vi "MEASURE_hysteresis - test.vi"() -> ()   [LabVIEW 2020]
uses:
  <vilib>/Utility/file.llb/Write To Spreadsheet File (DBL).vi
  <instrlib>/Keithley 24XX/Keithley 24XX.lvlib
panel:
  in  "Parameter":u16(ring)=1 items=["X", "Y", "R", "Theta", "Xh1", "Yh1", "Rh1", "Theta h1", "Xh2", "Yh2", "Rh2", "Theta h2", "Noise", "A1", "A2", "A3", "A4", "Frequency"]
  in  "harmonic 1":u8
  in  "Manual Phase":dbl=0.05
  in  "Sine Output Amplitude (1 V) 2":dbl=0.05
  in  "Input Connection (0: Single-Ended)":u16(ring) items=["Single-Ended Voltage", "Differential Voltage", "1 MOhm Current Gain", "100 MOhm Current Gain"]
  in  "frequency":dbl=50.0 format="%#_13g"
  out "loop run":i32
  in  "loop #":i32
  in  "Save data or not":bool=TRUE
  in  "path (folder + filename)":string="D:\\Kedar\\MoS2\\jw7_DJ_bulk_111213\\VvsHtr\\VvsHtr_300K"
  in  "Clear Plot":bool
  out "XY Graph":cluster{dbl[], dbl[]}(graph)
  out "LOCKIN Measurement":dbl
  out "gate voltage":dbl format="%#_13g"
  out "gate leaking":string="defbuffer1"
  in  "GATE STEP(mv)":i32
  in  "GATE Low Value (default 0)":dbl=1.0
  in  "GATE High Value":dbl=1.0
  in  "Function (0: Volts) 2":u16(ring) items=["Volts", "Current", "Resistance"]
  in  "Source Compaliance":dbl=1e-06
  in  "V address":refnum<visa-resource-name>="GPIB0::24::INSTR"
  in  "SD stabilization(S) 2":dbl format="%#_13g"
  in  "GATE / SD stablization 3":dbl format="%#_13g"
  in  "LOCKIN address":refnum<visa-resource-name>="GPIB0::24::INSTR"
  # "Lock-in"
  # "Gate Setting"
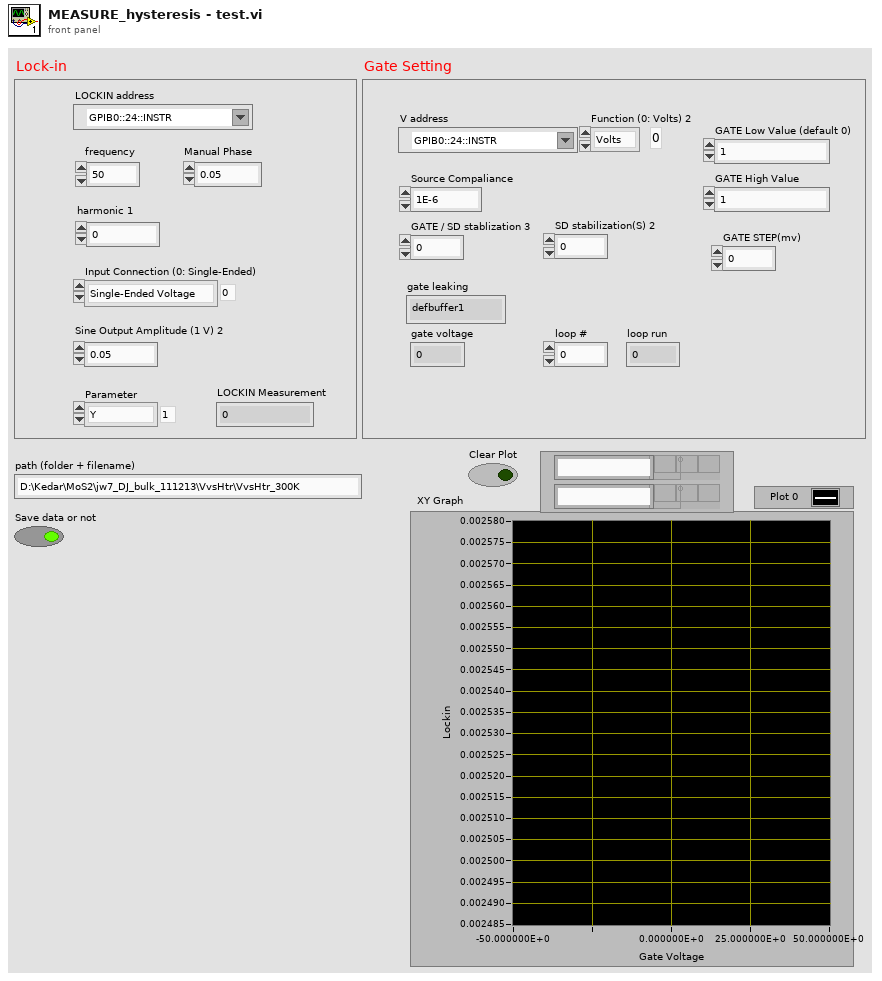
[diagram p1: front panel]
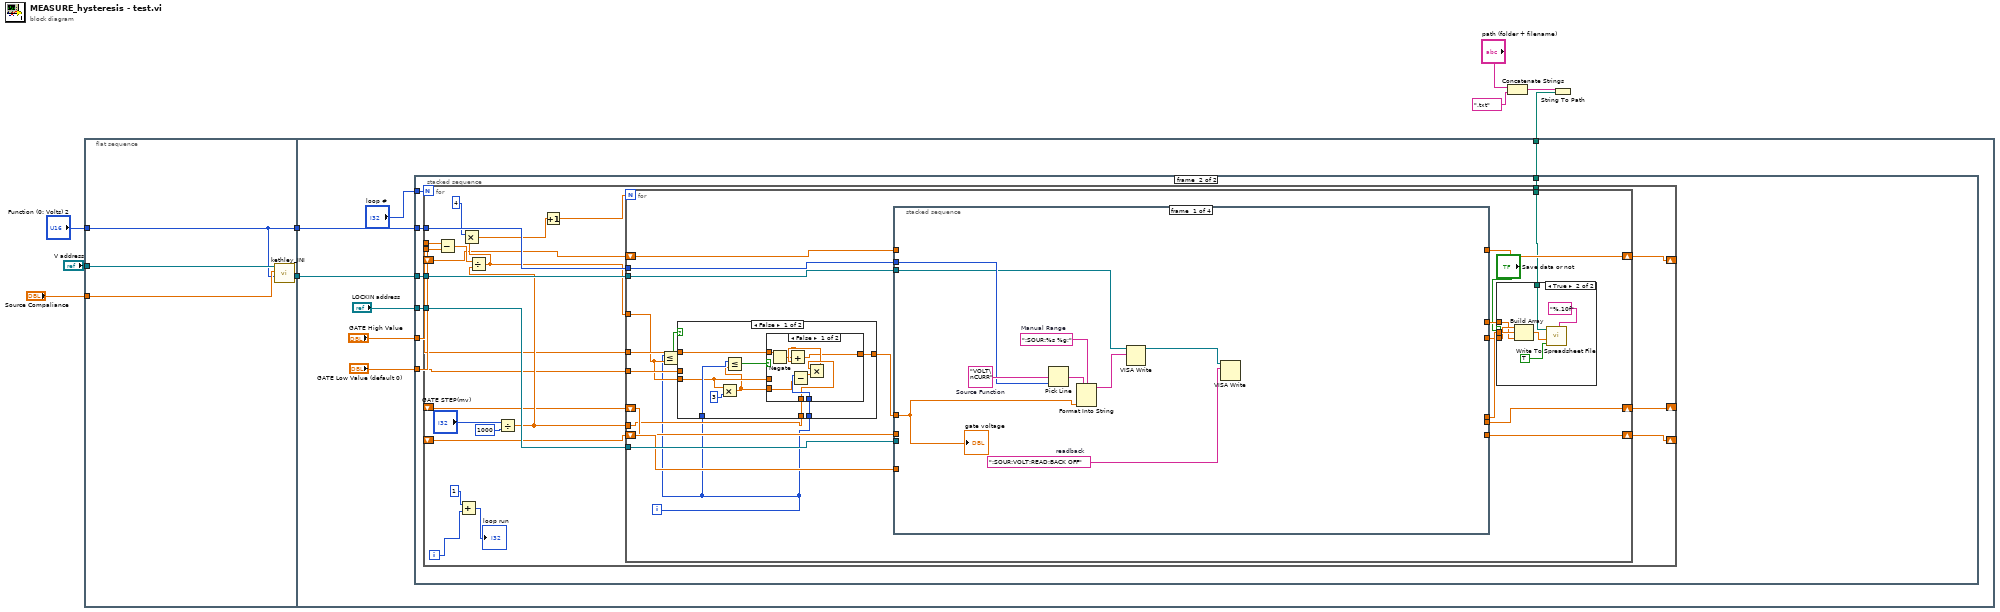
[diagram p0: block diagram]
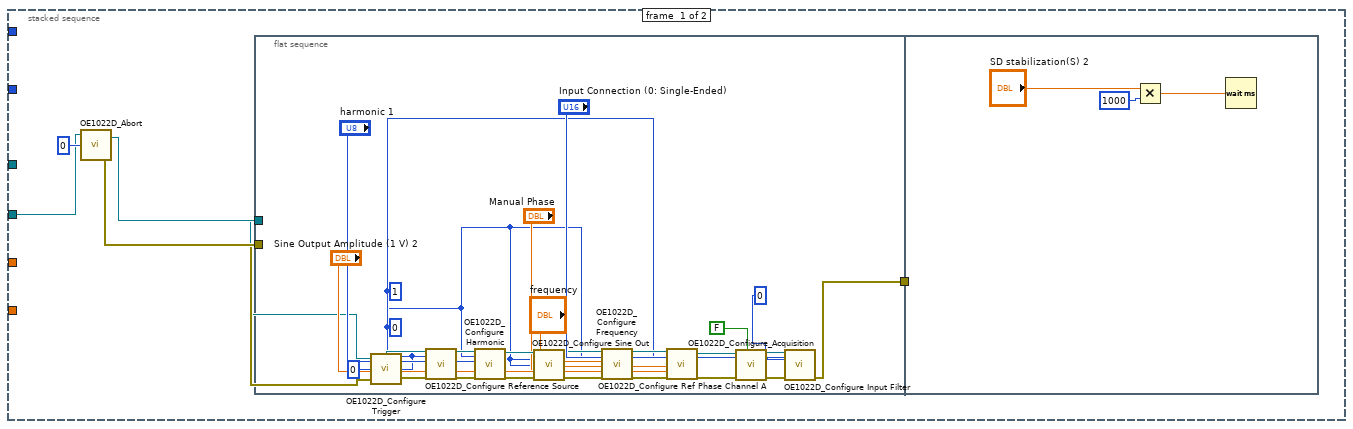
[diagram p2: hidden frame]
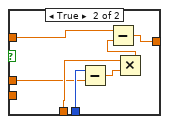
[diagram p4: hidden frame]
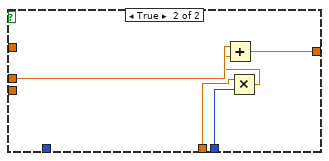
[diagram p5: hidden frame]
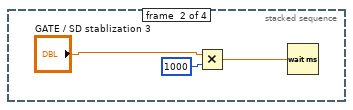
[diagram p6: hidden frame]
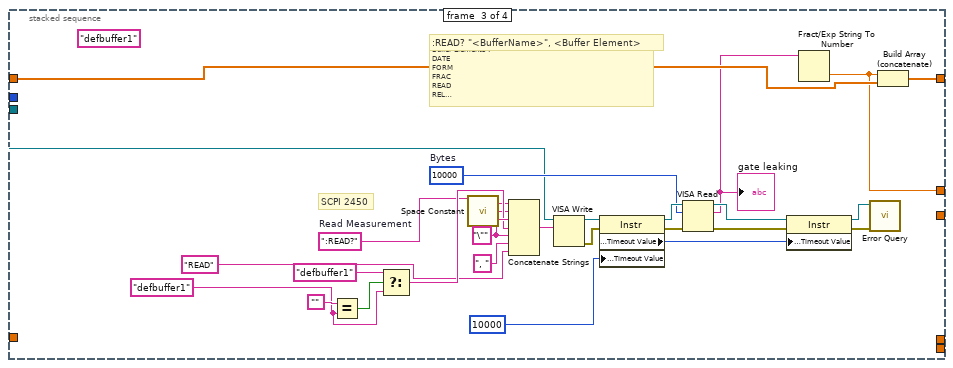
[diagram p7: hidden frame]
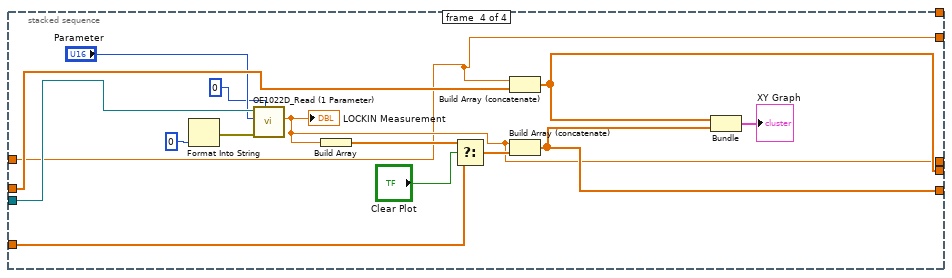
[diagram p8: hidden frame]
diagram:
  n1 = flat-sequence {
    tunnel: "V address" -> [w13]
    tunnel: "Source Compaliance" -> [w12]
    tunnel: "Function (0: Volts) 2" -> [w10]
    tunnel: [w11] -> w6
    tunnel: [w10] -> w5
    tunnel: w6 -> [w19]
    tunnel: w5 -> [w18]
    tunnel: w1 -> [w15]
    frame #0 {
      n2 = call "kethley_INI.vi"("Function (0: Volts) in"=w10, "Source Compaliance"=w12, "VISA Refnum in"=w13) -> ("VISA resource name out"=w11:refnum<visa-resource-name>)  [unwired: 8 in]
    }
    frame #1 {
      n3 = stacked-sequence {
        tunnel: "LOCKIN address" -> [w23 w60]
        tunnel: w19 -> [_ w61]
        tunnel: w18 -> [_ w62]
        tunnel: "GATE High Value" -> [_ w58]
        tunnel: "GATE Low Value (default 0)" -> [_ w59]
        tunnel: w15 -> [_ w57]
        tunnel: "loop #" -> [_ w56]
        frame #0 {
          n4 = call <instrlib>:"OE1022D_Abort.vi"("OE1022D A/B"=0, "VISA resource name"=w23) -> ("error out"=w22:errorcluster, "VISA resource name out"=w21:refnum<visa-resource-name>)  [unwired: 1 in]
          n5 = flat-sequence {
            tunnel: w21 -> [w27]
            tunnel: w22 -> [w28]
            tunnel: [w26] -> w25
            tunnel: w25 -> [_]
            frame #0 {
              w30 = 0
              w29 = 0
              w34 = 1
              n6 = call <instrlib>:"OE1022D_Configure Trigger.vi"("OE1022D A/B"=w29, "error in (no error)"=w28, "Trigger Source (0: Internal)"=0, "VISA resource name"=w27) -> ("error out"=w46:errorcluster, "VISA resource name out"=w47:refnum<visa-resource-name>)
              n7 = call <instrlib>:"OE1022D_Configure Reference Source.vi"("VISA resource name"=w47, "OE1022D A/B"=w29, "Reference Source"=w34, "error in (no error)"=w46) -> ("VISA resource name out"=w45:refnum<visa-resource-name>, "error out"=w43:errorcluster)  [unwired: 14 in]
              n8 = call <instrlib>:"OE1022D_Configure Harmonic.vi"("VISA resource name"=w45, "OE1022D A/B"=w29, "Harmonic 1"="harmonic 1", "error in (no error)"=w43) -> ("VISA resource name out"=w44:refnum<visa-resource-name>, "error out"=w42:errorcluster)  [unwired: 14 in]
              n9 = call <instrlib>:"OE1022D_Configure Sine Out.vi"("VISA resource name"=w44, "SineOut Mode"=w29, "OE1022D A/B"=w29, "Sine Output Amplitude (V)"="Sine Output Amplitude (1 V) 2", "error in (no error)"=w42) -> ("VISA resource name out"=w50:refnum<visa-resource-name>, "error out"=w49:errorcluster)  [unwired: 9 in]
              n10 = call <instrlib>:"OE1022D_Configure Frequency.vi"("VISA resource name"=w50, "OE1022D A/B"=w29, "Internal Frequency(Hz)"="frequency", "error in (no error)"=w49) -> ("VISA resource name out"=w40:refnum<visa-resource-name>, "error out"=w35:errorcluster)  [unwired: 14 in]
              n11 = call <instrlib>:"OE1022D_Configure Ref Phase Channel A.vi"("VISA resource name"=w40, "Reference Source"=w34, "Internal Frequency(Hz)"="frequency", "Phase  (degree)"="Manual Phase", "error in (no error)"=w35) -> ("VISA resource name out"=w39:refnum<visa-resource-name>, "error out"=w36:errorcluster)  [unwired: 13 in]
              n12 = call <instrlib>:"OE1022D_Configure_Acquisition.vi"("Continuous Storage (T: Enable)"=FALSE, "error in (no error)"=w36, "OE1022D A/B"=w30, "VISA resource name"=w39) -> ("error out"=w37:errorcluster, "VISA resource name out"=w38:refnum<visa-resource-name>)  [unwired: 6 in]
              n13 = call <instrlib>:"OE1022D_Configure Input Filter.vi"("VISA resource name"=w38, "Input Source"="Input Connection (0: Single-Ended)", "OE1022D A/B"=w30, "error in (no error)"=w37) -> ("error out"=w26:errorcluster)  [unwired: 10 in, 1 out]
            }
            frame #1 {
              n14 = Multiply(x="SD stabilization(S) 2", y=1000) -> (x*y=w55:dbl)
              n15 = Wait (ms)(milliseconds to wait=w55) -> ()  [unwired: 1 out]
            }
          }
        }
        frame #1 {
          n16 = for {
            N: w56 -> [_]
            tunnel: w62 -> [w85]
            tunnel: w61 -> [w84]
            tunnel: w60 -> [w83]
            tunnel: w59 -> [w77]
            tunnel: w58 -> [w76]
            tunnel: w57 -> [w75]
            shift-right: [w71] -> _
            shift-left: _ -> [w70]
            shift-right: [w69] -> _
            shift-left: _ -> [w67]
            shift-right: [w68] -> _
            shift-left: _ -> [w66]
            i -> [w64]
            n17 = Subtract(x=w76, y=w77) -> (x-y=w79:dbl)
            n18 = Add(x=1, y=w64) -> (x+y=→"loop run":i32)
            n19 = Divide(x="GATE STEP(mv)", y=1000) -> (x/y=w78:dbl)
            n20 = Divide(x=w79, y=w78) -> (x/y=w74:dbl)
            n21 = Multiply(x=4, y=w74) -> (x*y=w73:dbl)
            n22 = Increment(x=w73) -> (x+1=w72:dbl)
            n23 = for {
              N: w72 -> [_]
              tunnel: w85 -> [w106]
              tunnel: w84 -> [w105]
              tunnel: w83 -> [w104]
              tunnel: w78 -> [w95]
              shift-right: [w103] -> w71
              shift-left: w70 -> [w102]
              shift-right: [w99] -> w68
              shift-left: w66 -> [w101]
              shift-right: [w98] -> w69
              shift-left: w67 -> [w100]
              tunnel: w74 -> [w92]
              tunnel: w77 -> [w96]
              tunnel: w76 -> [w93]
              tunnel: w75 -> [w87]
              i -> [w91]
              n24 = Less Or Equal?(x=w91, y=w92) -> (x <= y?=w97:bool)
              n25 = case shown="False" w97 {
                tunnel: w96 -> [_ w142]
                tunnel: w91 -> [w122 w141]
                tunnel: w95 -> [w121 w140]
                tunnel: [w119 w138] -> w94
                tunnel: w93 -> [w120 _]
                tunnel: w92 -> [w115 _]
                tunnel: w91 -> [w118 _]
                frame False {
                  n26 = Multiply(x=w115, y=3) -> (x*y=w114:dbl)
                  n27 = Less Or Equal?(x=w118, y=w114) -> (x <= y?=w116:bool)
                  n28 = case shown="False" w116 {
                    tunnel: w122 -> [w130 w137]
                    tunnel: w121 -> [w128 w135]
                    tunnel: w120 -> [w124 w133]
                    tunnel: [w126 w132] -> w119
                    tunnel: w115 -> [_ w131]
                    tunnel: w114 -> [w123 _]
                    frame False {
                      n29 = Negate(x=w124) -> (-x=w125:dbl)
                      n30 = Subtract(x=w130, y=w123) -> (x-y=w129:dbl)
                      n31 = Multiply(x=w128, y=w129) -> (x*y=w127:dbl)
                      n32 = Add(x=w125, y=w127) -> (x+y=w126:dbl)
                    }
                    frame True {
                      n33 = Subtract(x=w137, y=w131) -> (x-y=w136:dbl)
                      n34 = Multiply(x=w135, y=w136) -> (x*y=w134:dbl)
                      n35 = Subtract(x=w133, y=w134) -> (x-y=w132:dbl)
                    }
                  }
                }
                frame True {
                  n36 = Multiply(x=w140, y=w141) -> (x*y=w139:dbl)
                  n37 = Add(x=w142, y=w139) -> (x+y=w138:dbl)
                }
              }
              n38 = stacked-sequence {
                tunnel: w106 -> [w147 _ _ _]
                tunnel: w105 -> [w146 _ w159 _]
                tunnel: w104 -> [_ _ _ w186]
                tunnel: w94 -> [w145 _ _ w184]
                tunnel: [_ _ w157 _] -> w103
                tunnel: w102 -> [_ _ w158 _]
                tunnel: w101 -> [_ _ _ w190]
                tunnel: w100 -> [_ _ _ w187]
                tunnel: [_ _ _ w189] -> w99
                tunnel: [_ _ _ w188] -> w98
                tunnel: [_ _ _ w185] -> w90
                tunnel: [_ _ _ w184] -> w89
                tunnel: [_ _ w155 _] -> w88
                frame #0 {
                  w143 = ":SOUR:VOLT:READ:BACK OFF"  # readback
                  w149 = "VOLT\nCURR"  # Source Function
                  w150 = ":SOUR:%s %g;"  # Manual Range
                  n39 = Pick Line(multi-line string=w149, line index=w147) -> (output string=w148:string)  [unwired: 1 out]
                  n40 = Format Into String(format string=w150, w148, w145) -> (resulting string=w151:string)  [unwired: 2 in, 1 out]
                  n41 = VISA Write(VISA resource name=w146, write buffer=w151) -> (VISA resource name out=w144:refnum<visa-resource-name>)  [unwired: 1 in, 2 out]
                  n42 = VISA Write(VISA resource name=w144, write buffer=w143) -> ()  [unwired: 1 in, 3 out]
                  "gate voltage" <- w145
                }
                frame #1 {
                  n43 = Multiply(x="GATE / SD stablization 3", y=1000) -> (x*y=w154:dbl)
                  n44 = Wait (ms)(milliseconds to wait=w154) -> ()  [unwired: 1 out]
                }
                frame #2 {
                  w170 = "defbuffer1" ("Buffer Name (defbuffer1) 2")
                  (unwired) "defbuffer1" ("t")
                  w168 = "\""
                  w165 = ":READ?"  # Read Measurement
                  w174 = u32 10000  # Bytes
                  # "NOTE :\nBuffer Elements :\nDATE\nFORM\nFRAC\nREAD\nREL\nSEC\nSOUR\nSOURFORM\nSOURSTAT\nSOURUNIT\nSTAT\nTIME\nTsT\nUNIT"
                  # ":READ? \"<BufferName>\", <Buffer Element>"
                  # "SCPI 2450"
                  n45 = Equal?(x="", y=w170) -> (x = y?=w171:bool)
                  n46 = Select(t="defbuffer1", s=w171, f=w170) -> (s? t:f=w167:string)
                  n47 = call <vilib>:"Space Constant.vi"() -> ("String"=w166:string)
                  n48 = Concatenate Strings(w165, w166, w168, w167, w168, ", " ("string"), "READ" ("Buffer Elements 2")) -> (w181:string)
                  n49 = VISA Write(VISA resource name=w159, write buffer=w181) -> (VISA resource name out=w173:refnum<visa-resource-name>, error out=w180:errorcluster)  [unwired: 1 in, 1 out]
                  n50 = property class="Instr"(reference=w173, error in=w180, "General Settings:Timeout Value"=10000 ("Timeout (10000 ms) 2")) -> (reference out=w179:refnum<visa-resource-name>, error out=w178:errorcluster, "General Settings:Timeout Value"=w175:u32)
                  n51 = VISA Read(VISA resource name=w179, byte count=w174, error in (no error)=w178) -> (VISA resource name out=w177:refnum<visa-resource-name>, read buffer=w156:string, error out=w176:errorcluster)  [unwired: 1 out]
                  "gate leaking" <- w156
                  n52 = property class="Instr"(reference=w177, error in=w176, "General Settings:Timeout Value"=w175) -> (reference out=w163:refnum<visa-resource-name>, error out=w162:errorcluster)
                  n53 = Fract/Exp String To Number(string=w156) -> (number=w155:dbl)  [unwired: 3 in, 1 out]
                  n54 = call <instrlib>:"Error Query.vi"("error in (no error)"=w162, "VISA resource name"=w163) -> ()  [unwired: 6 in, 4 out]
                  n55 = Build Array (concatenate)(w155, w158) -> (w157:dbl[])
                }
                frame #3 {
                  n56 = Format Into String(0) -> (error out=w196:errorcluster)  [unwired: 3 in, 1 out]
                  n57 = call <instrlib>:"OE1022D_Read (1 Parameter).vi"("OE1022D A/B"=0, "error in (no error)"=w196, "Parameter"="Parameter", "VISA resource name"=w186) -> ("Measurement"=w185:dbl)  [unwired: 5 in, 2 out]
                  "LOCKIN Measurement" <- w185
                  n58 = Build Array(w185) -> (w193:dbl[])
                  n59 = Select(t=w193, s="Clear Plot", f=w190) -> (s? t:f=w194:dbl[])
                  n60 = Build Array (concatenate)(w184, w187) -> (w188:dbl[])
                  n61 = Build Array (concatenate)(w185, w194) -> (w189:dbl[])
                  n62 = Bundle(w188, w189) -> (→"XY Graph":cluster{dbl[], dbl[]})  [unwired: 1 in]
                }
              }
              n63 = case shown="True" "Save data or not" {
                tunnel: w90 -> [_ w113]
                tunnel: w89 -> [_ w112]
                tunnel: w88 -> [_ w111]
                tunnel: w87 -> [_ w109]
                frame False {
                }
                frame True {
                  n64 = Build Array(w112, w113, w111) -> (w110:dbl[])
                  n65 = call-poly <vilib>:"Write To Spreadsheet File.vi"("format (%.3f)"="%.10f", "append to file? (new file:F)"=TRUE, "1D data"=w110, "file path (dialog if empty)"=w109) -> ()  [unwired: 4 in, 1 out]
                }
              }
            }
          }
        }
      }
    }
  }
  n66 = Concatenate Strings("path (folder + filename)", ".txt") -> (w2:string)
  n67 = String To Path(string=w2) -> (path=w1:path)
